vi "Load_Cycle_ON_OFF.vi"(0 "SI804.lvclass in":refnum<class "SI804.lvclass">, 7 "3 JSA30 DG606\nXA01":bool, 11 "error in":errorcluster) -> (4 "SI804.lvclass out":refnum<class "SI804.lvclass">, 8 "Load-cycle Puls":bool, 15 "error out":errorcluster)   [LabVIEW 2022 SP3, in "SI804.lvclass"]
uses:
  SI804.lvclass
  SI804.lvclass/SI804.ctl
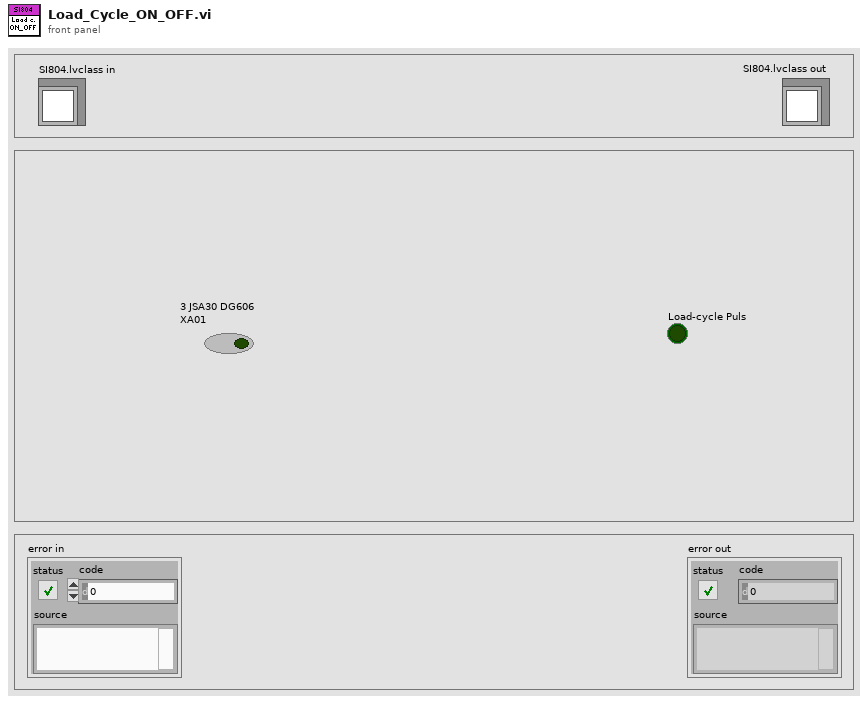
[diagram p1: front panel]
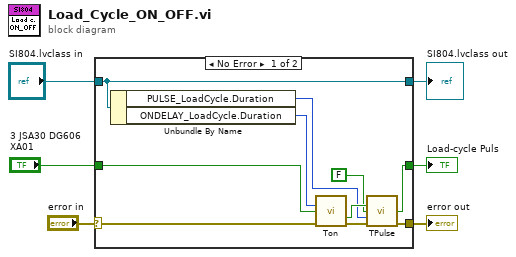
[diagram p0: block diagram]
diagram:
  n1 = case shown="No Error" "error in" {
    selector: "error in" -> [w9 w18]
    tunnel: "3 JSA30 DG606\nXA01" -> [w16 _]
    tunnel: "SI804.lvclass in" -> [w10 w17]
    tunnel: [w11 _] -> w4
    tunnel: [w10 w17] -> w3
    tunnel: [w7 w18] -> w1
    frame No Error {
      n2 = Unbundle By Name(w10) -> ("PULSE_LoadCycle.Duration"=w13:i32, "ONDELAY_LoadCycle.Duration"=w14:i32)
      n3 = call "Ton.vi"("Ton"=w14, "input"=w16, "error in"=w9) -> ("Binary out"=w15:bool, "error out"=w8:errorcluster)  [unwired: 8 in, 3 out]
      n4 = call "TPulse.vi"("trigger"=w15, "Reset"=FALSE, "TPulse"=w13, "error in"=w8) -> ("output"=w11:bool, "error out"=w7:errorcluster)  [unwired: 9 in, 1 out]
    }
    frame Error {
    }
  }
  "Load-cycle Puls" <- w4
  "SI804.lvclass out" <- w3
  "error out" <- w1
